vi "Peregrine_read_temperature.vi"(0 "Handle in":refnum<visa-resource-name>, 2 "Address":u8, 5 "i2c address":u32, 11 "error":errorcluster) -> (3 "Address response":u8, 4 "Handle out":refnum<visa-resource-name>, 6 "Key response":u32, 8 "Value response":i32, 10 "Decoded value":dbl, 15 "error out":errorcluster)   [LabVIEW 2019]
panel:
  out "Command":i32
  # "Inputs"
  # "Response message"
  # "Output"
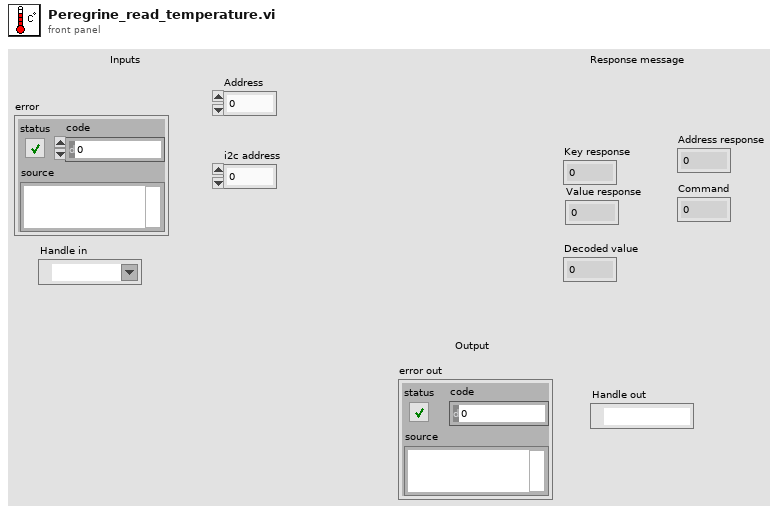
[diagram p1: front panel]
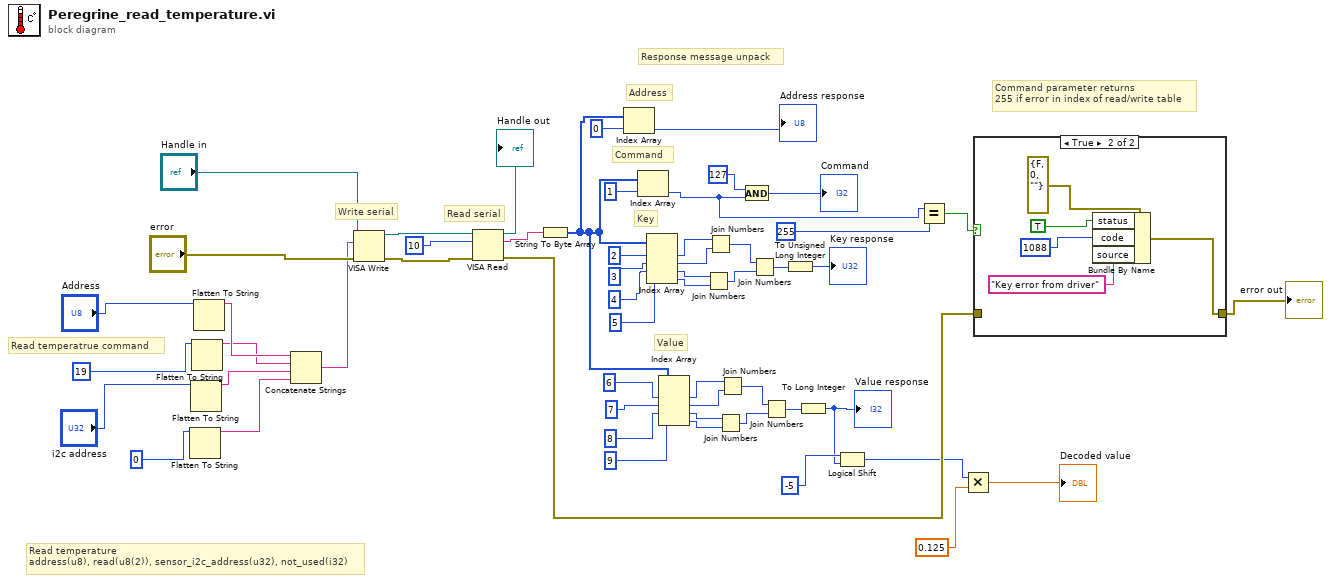
[diagram p0: block diagram]
diagram:
  # "Command parameter returns\n255 if error in index of read/write table"
  # "Value"
  # "Response message unpack"
  # "Read temperatrue command"
  # "Command"
  # "Address"
  # "Key"
  # "Read serial"
  # "Write serial"
  # "Read temperature\naddress(u8), read(u8(2)), sensor_i2c_address(u32), not_used(i32)"
  n1 = Flatten To String(anything=0) -> (data string=w29:string)  [unwired: 3 in, 2 out]
  n2 = Flatten To String(anything="i2c address") -> (data string=w30:string)  [unwired: 3 in, 2 out]
  n3 = Flatten To String(anything=u8 19) -> (data string=w2:string)  [unwired: 3 in, 2 out]
  n4 = Flatten To String(anything="Address") -> (data string=w32:string)  [unwired: 3 in, 2 out]
  n5 = Concatenate Strings(w32, w2, w30, w29) -> (w1:string)
  n6 = VISA Write(VISA resource name="Handle in", write buffer=w1, error in (no error)="error") -> (VISA resource name out=w55:refnum<visa-resource-name>, error out=w34:errorcluster)  [unwired: 1 out]
  n7 = VISA Read(VISA resource name=w55, byte count=10, error in (no error)=w34) -> (VISA resource name out=→"Handle out":refnum<visa-resource-name>, read buffer=w53:string, error out=w10:errorcluster)  [unwired: 1 out]
  n8 = String To Byte Array(string=w53) -> (unsigned byte array=w20:u8[])
  n9 = Index Array(array=w20, index=0) -> (element=→"Address response":u8)
  n10 = Index Array(array=w20, index=1) -> (element=w13:u8)
  n11 = Index Array(array=w20, index #1=2, index #2=3, index #3=4, index #4=5) -> (element #1=w46:u8, element #2=w45:u8, element #3=w44:u8, element #4=w43:u8)
  n12 = Index Array(array=w20, index #1=6, index #2=7, index #3=8, index #4=9) -> (element #1=w27:u8, element #2=w26:u8, element #3=w25:u8, element #4=w24:u8)
  n13 = Join Numbers(hi=w44, lo=w43) -> ((hi.lo)=w42:u16)
  n14 = Join Numbers(hi=w46, lo=w45) -> ((hi.lo)=w41:u16)
  n15 = Join Numbers(hi=w25, lo=w24) -> ((hi.lo)=w23:u16)
  n16 = Join Numbers(hi=w27, lo=w26) -> ((hi.lo)=w22:u16)
  n17 = And(x=127, y=w13) -> (x .and. y?=→"Command":i32)
  n18 = Join Numbers(hi=w41, lo=w42) -> ((hi.lo)=w15:u32)
  n19 = Join Numbers(hi=w22, lo=w23) -> ((hi.lo)=w16:u32)
  n20 = To Unsigned Long Integer(number=w15) -> (unsigned 32bit integer=→"Key response":u32)
  n21 = To Long Integer(number=w16) -> (32bit integer=w6:i32)
  "Value response" <- w6
  n22 = Logical Shift(y=-5, x=w6) -> (x << y=w4:i32)
  n23 = Equal?(x=w13, y=255) -> (x = y?=w11:bool)
  n24 = Multiply(x=w4, y=0.125) -> (x*y=→"Decoded value":dbl)
  n25 = case shown="True" w11 {
    tunnel: w10 -> [w56 _]
    tunnel: [w56 w58] -> w9
    frame False {
    }
    frame True {
      n26 = Bundle By Name(cluster=errorcluster {"status"=FALSE, "code"=0, "source"=""} ("error constant"), "status"=TRUE, "code"=1088, "source"="Key error from driver") -> (w58:errorcluster)
    }
  }
  "error out" <- w9
